vi "CRYRub & Buzz Pe[k,n].vi"(0 "Real matrix":dbl[][](array[numeric]), 1 "Version":i32, 2 "size":i32, 3 "Fsp[k]":dbl[](array[numeric])) -> (5 "Pe[k]":dbl[](array[numeric]))   [LabVIEW 2013]
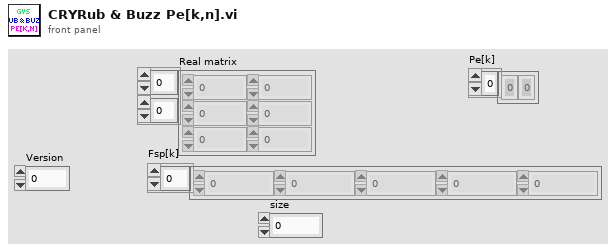
[diagram p1: front panel]
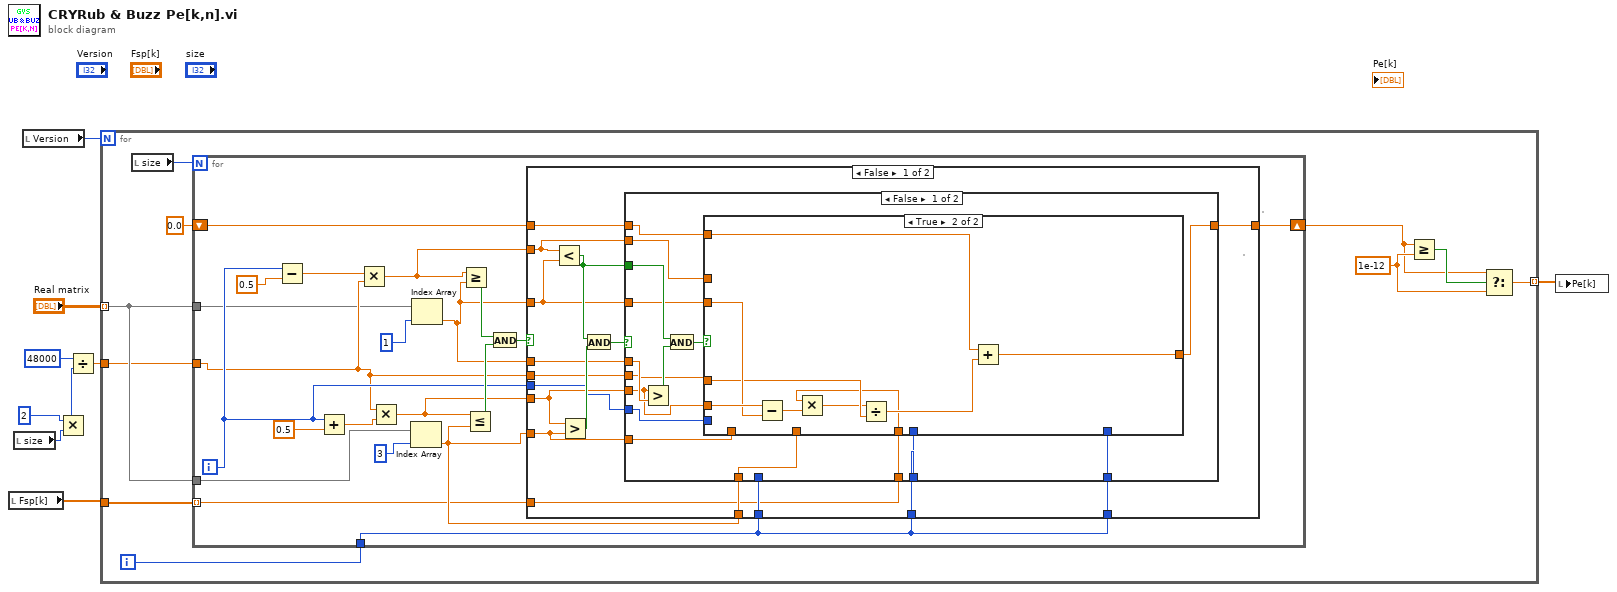
[diagram p0: block diagram]
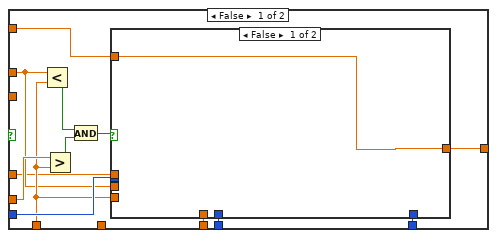
[diagram p2: hidden frame]
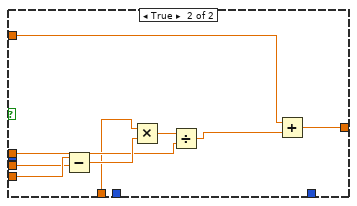
[diagram p3: hidden frame]
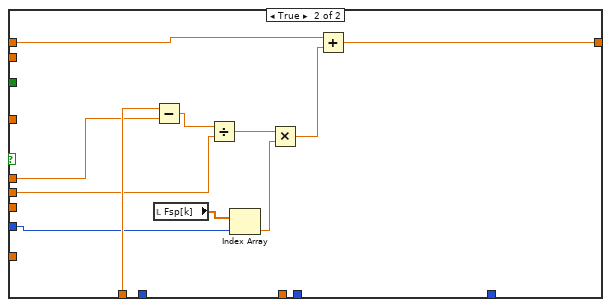
[diagram p4: hidden frame]
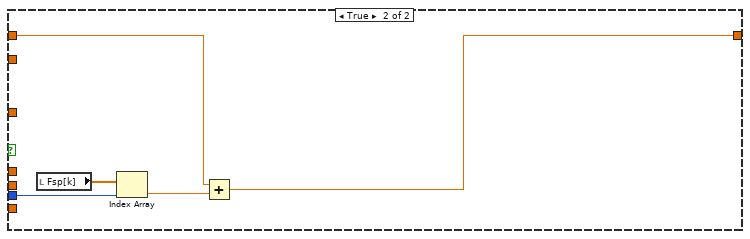
[diagram p5: hidden frame]
diagram:
  n1 = local read "Fsp[k]"() -> (w2:dbl[])
  n2 = local read "size"() -> (w4:i32)
  n3 = local read "Version"() -> (w6:i32)
  n4 = Multiply(x=2, y=w4) -> (x*y=w3:i32)
  n5 = Divide(x=48000, y=w3) -> (x/y=w8:dbl)
  n6 = for {
    N: w6 -> [_]
    tunnel: "Real matrix" -> [w18] mode=indexing
    tunnel: w8 -> [w17]
    tunnel: w2 -> [w14]
    tunnel: [w10] -> w1 mode=indexing
    i -> [w19]
    w13 = 1e-12
    n7 = local read "size"() -> (w16:i32)
    n8 = for {
      N: w16 -> [_]
      tunnel: w19 -> [w25]
      tunnel: w18 -> [w29]
      tunnel: w18 -> [w26]
      tunnel: w17 -> [w30]
      shift-right: [w22] -> w11
      shift-left: 0.0 -> [w21]
      tunnel: w14 -> [w20] mode=indexing
      i -> [w31]
      n9 = Subtract(x=w31, y=0.5) -> (x-y=w39:dbl)
      n10 = Add(x=w31, y=0.5) -> (x+y=w37:dbl)
      n11 = Multiply(x=w39, y=w30) -> (x*y=w33:dbl)
      n12 = Multiply(x=w30, y=w37) -> (x*y=w32:dbl)
      n13 = Index Array(array=w26, index=3) -> (element=w27:dbl)
      n14 = Index Array(array=w29, index=1) -> (element=w28:dbl)
      n15 = Greater Or Equal?(x=w33, y=w28) -> (x >= y?=w36:bool)
      n16 = Less Or Equal?(x=w32, y=w27) -> (x <= y?=w35:bool)
      n17 = And(x=w36, y=w35) -> (x .and. y?=w34:bool)
      n18 = case shown="False" w34 {
        tunnel: w25 -> [w55 _]
        tunnel: w33 -> [w46 _]
        tunnel: w28 -> [w47 _]
        tunnel: w32 -> [w49 _]
        tunnel: w27 -> [w45 _]
        tunnel: w27 -> [w54 _]
        tunnel: w28 -> [w53 _]
        tunnel: w30 -> [w52 _]
        tunnel: w31 -> [w51 w121]
        tunnel: w25 -> [w50 _]
        tunnel: w25 -> [w44 _]
        tunnel: [w42 w118] -> w22
        tunnel: w21 -> [w43 w117]
        tunnel: w20 -> [w41 _]
        frame False {
          n19 = Less?(x=w46, y=w47) -> (x < y?=w48:bool)
          n20 = Greater?(x=w49, y=w45) -> (0:w57:bool)
          n21 = And(x=w48, y=w57) -> (x .and. y?=w56:bool)
          n22 = case shown="False" w56 {
            tunnel: w55 -> [_ _]
            tunnel: w54 -> [w58 w116]
            tunnel: w53 -> [w73 w115]
            tunnel: w52 -> [w67 w113]
            tunnel: w51 -> [w66 w109]
            tunnel: w50 -> [w65 _]
            tunnel: w49 -> [w69 _]
            tunnel: w48 -> [w72 _]
            tunnel: w47 -> [w68 _]
            tunnel: w46 -> [w64 _]
            tunnel: w45 -> [w63 _]
            tunnel: w44 -> [w62 _]
            tunnel: w43 -> [w61 w107]
            tunnel: [w60 w106] -> w42
            tunnel: w41 -> [w59 _]
            frame False {
              n23 = Greater?(x=w69, y=w73) -> (0:w71:bool)
              n24 = And(x=w72, y=w71) -> (x .and. y?=w70:bool)
              n25 = case shown="True" w70 {
                tunnel: w69 -> [w86 w105]
                tunnel: w68 -> [_ w104]
                tunnel: w67 -> [w79 w103]
                tunnel: w66 -> [w82 _]
                tunnel: w65 -> [w78 _]
                tunnel: w64 -> [w80 _]
                tunnel: w63 -> [w81 _]
                tunnel: w62 -> [w77 _]
                tunnel: w61 -> [w76 w99]
                tunnel: [w75 w98] -> w60
                tunnel: w59 -> [w74 w97]
                tunnel: w58 -> [_ _]
                frame False {
                  n26 = Less?(x=w80, y=w81) -> (x < y?=w85:bool)
                  n27 = Greater?(x=w86, y=w81) -> (0:w84:bool)
                  n28 = And(x=w85, y=w84) -> (x .and. y?=w83:bool)
                  n29 = case shown="False" w83 {
                    tunnel: w82 -> [_ _]
                    tunnel: w81 -> [_ w96]
                    tunnel: w80 -> [_ w95]
                    tunnel: w79 -> [_ w92]
                    tunnel: w78 -> [_ _]
                    tunnel: w77 -> [_ _]
                    tunnel: w76 -> [w87 w89]
                    tunnel: [w87 w88] -> w75
                    tunnel: w74 -> [_ w90]
                    frame False {
                    }
                    frame True {
                      n30 = Subtract(x=w96, y=w95) -> (x-y=w94:dbl)
                      n31 = Multiply ("Multiply.vi")(x=w90, y=w94) -> (x*y=w93:dbl)
                      n32 = Divide(x=w93, y=w92) -> (x/y=w91:dbl)
                      n33 = Add ("Add.vi")(x=w89, y=w91) -> (x+y=w88:dbl)
                    }
                  }
                }
                frame True {
                  n34 = Subtract ("Subtract.vi")(x=w105, y=w104) -> (x-y=w102:dbl)
                  n35 = Multiply ("Multiply.vi")(x=w97, y=w102) -> (x*y=w101:dbl)
                  n36 = Divide(x=w101, y=w103) -> (x/y=w100:dbl)
                  n37 = Add ("Add.vi")(x=w99, y=w100) -> (x+y=w98:dbl)
                }
              }
            }
            frame True {
              n38 = Subtract ("Subtract.vi")(x=w116, y=w115) -> (x-y=w112:dbl)
              n39 = local read "Fsp[k]"() -> (w110:dbl[])
              n40 = Divide(x=w112, y=w113) -> (x/y=w111:dbl)
              n41 = Index Array(array=w110, index=w109) -> (element=w108:dbl)
              n42 = Multiply ("Multiply.vi")(x=w111, y=w108) -> (x*y=w114:dbl)
              n43 = Add ("Add.vi")(x=w107, y=w114) -> (x+y=w106:dbl)
            }
          }
        }
        frame True {
          n44 = local read "Fsp[k]"() -> (w119:dbl[])
          n45 = Index Array(array=w119, index=w121) -> (element=w120:dbl)
          n46 = Add ("Add.vi")(x=w117, y=w120) -> (x+y=w118:dbl)
        }
      }
    }
    n47 = Greater Or Equal?(x=w11, y=w13) -> (x >= y?=w12:bool)
    n48 = Select(t=w11, s=w12, f=w13) -> (s? t:f=w10:dbl)
  }
  n49 = local write "Pe[k]"(w1) -> ()
